vi "EncoderPacketParser.vi"(4 "Message":u8[](array[numeric])) -> (1 "encoderPacket":T1 {"Encoder Count" format="%#_6f"})   [LabVIEW 2014]
uses:
  EncoderPacket.ctl
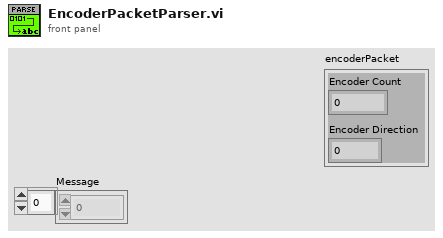
[diagram p1: front panel]
types:
  T1 = typedef "EncoderPacket.ctl" = cluster{"Encoder Count":dbl, "Encoder Direction":dbl}
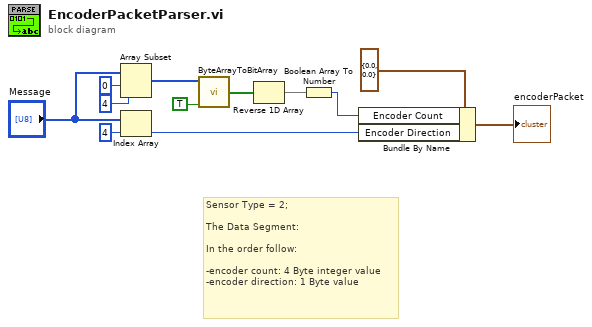
[diagram p0: block diagram]
diagram:
  # "Sensor Type = 2;\n\nThe Data Segment:\n\nIn the order follow:\n\n-encoder count: 4 Byte integer value\n-encoder direction: 1 Byte value"
  n1 = Array Subset(array="Message", index=0, length=4) -> (w2:u8[])
  n2 = Index Array(array="Message", index=4) -> (element=w6:u8)
  n3 = call "ByteArrayToBitArray.vi"("Flip Endian"=TRUE, "Byte Array In"=w2) -> ("Bit Array Out"=w1:bool[])  [unwired: 4 in]
  n4 = Reverse 1D Array(array=w1) -> (reversed array=w4:bool[])
  n5 = Boolean Array To Number(Boolean array=w4) -> (number=w5:u32)
  n6 = Bundle By Name(cluster=T1 {"Encoder Count"=0.0, "Encoder Direction"=0.0} ("encoderPacket"), "Encoder Count"=w5, "Encoder Direction"=w6) -> (→"encoderPacket":T1)
